vi "Calculate Scan Start and Frequency.vi"(9 "Start delay (s)":u16, 10 "Start offset (fraction)":dbl, 11 "Scan Period (uS)":u32) -> (2 "Start time":timestamp, 3 "Frequency":dbl)   [LabVIEW 2015, in "NI Synchronization Engine.lvlib"]
uses:
  NI Synchronization Engine.lvlib
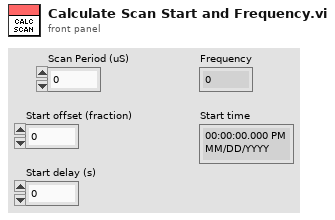
[diagram p1: front panel]
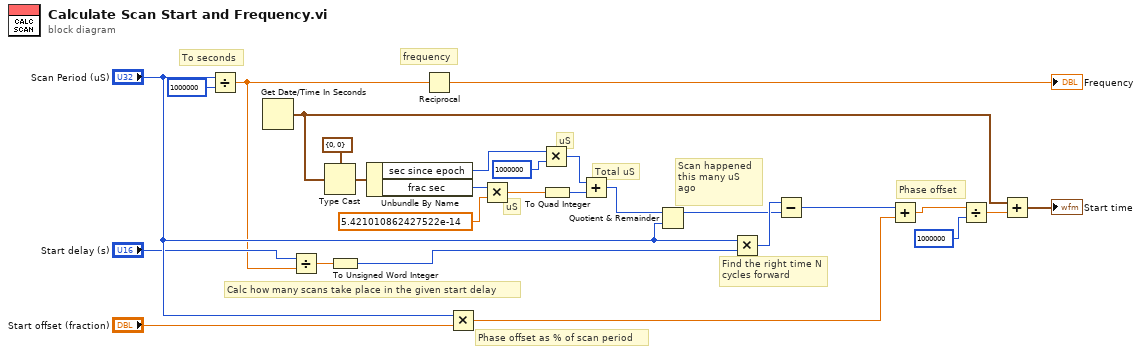
[diagram p0: block diagram]
diagram:
  # "Scan happened this many uS ago"
  # "Calc how many scans take place in the given start delay"
  # "Phase offset as % of scan period"
  # "Phase offset"
  # "Find the right time N cycles forward"
  # "Total uS"
  # "uS"
  # "uS"
  # "To seconds"
  # "frequency"
  n1 = Divide(x="Scan Period (uS)", y=u32 1000000) -> (x/y=w3:dbl)
  n2 = Get Date/Time In Seconds() -> (seconds since 1Jan1904=w6:timestamp)
  n3 = Divide(x="Start delay (s)", y=w3) -> (x/y=w2:dbl)
  n4 = Type Cast(type=cluster{"sec since epoch":i64, "frac sec":u64} {"sec since epoch"=0, "frac sec"=0}, x=w6) -> (*(type *) &x=w15:cluster{"sec since epoch":i64, "frac sec":u64})
  n5 = To Unsigned Word Integer(number=w2) -> (unsigned 16bit integer=w1:u16)
  n6 = Unbundle By Name(w15) -> ("sec since epoch"=w11:i64, "frac sec"=w14:u64)
  n7 = Reciprocal(x=w3) -> (1/x=→"Frequency":dbl)
  n8 = Multiply(x="Scan Period (uS)", y="Start offset (fraction)") -> (x*y=w25:dbl)
  n9 = Multiply(x=w14, y=5.421010862427522e-14) -> (x*y=w10:dbl)
  n10 = Multiply(x=w11, y=i64 1000000) -> (x*y=w13:i64)
  n11 = To Quad Integer(1:w10) -> (0:w12:i64)
  n12 = Add(x=w13, y=w12) -> (x+y=w5:i64)
  n13 = Quotient & Remainder(x=w5, y="Scan Period (uS)") -> (x-y*floor(x/y)=w19:i64)  [unwired: 1 out]
  n14 = Multiply(x="Scan Period (uS)", y=w1) -> (x*y=w23:u32)
  n15 = Subtract(x=w23, y=w19) -> (x-y=w20:i64)
  n16 = Add(x=w20, y=w25) -> (x+y=w24:dbl)
  n17 = Divide(x=w24, y=u64 1000000) -> (x/y=w22:dbl)
  n18 = Add(x=w6, y=w22) -> (x+y=→"Start time":timestamp)
